vi "Close.vi"(8 "error in (no error)":errorcluster, 11 "Inst.FP in":refnum<class "Inst.FP.lvclass">) -> (0 "error out":errorcluster, 3 "Inst.FP out":refnum<class "Inst.FP.lvclass">)   [LabVIEW 2019, in "Inst.FP.lvclass"]
uses:
  Inst.FP.lvclass
  <userlib>/LevyLab/Instrument Framework/Instrument/Instrument.lvclass
  <userlib>/LevyLab/Instrument Framework/Instrument Types/Cryostat/Instrument.Cryostat.lvclass
  C:/Program Files (x86)/National Instruments/LabVIEW 2019/user.lib/LevyLab/Instrument Framework/Instrument Types/Cryostat/Instrument.Cryostat.lvclass
  C:/Program Files (x86)/National Instruments/LabVIEW 2019/user.lib/LevyLab/Instrument Framework/Instrument/Instrument.lvclass
  C:/Program Files (x86)/National Instruments/LabVIEW 2019/vi.lib/JKI/JKI SMO/SMO/SMO.lvclass
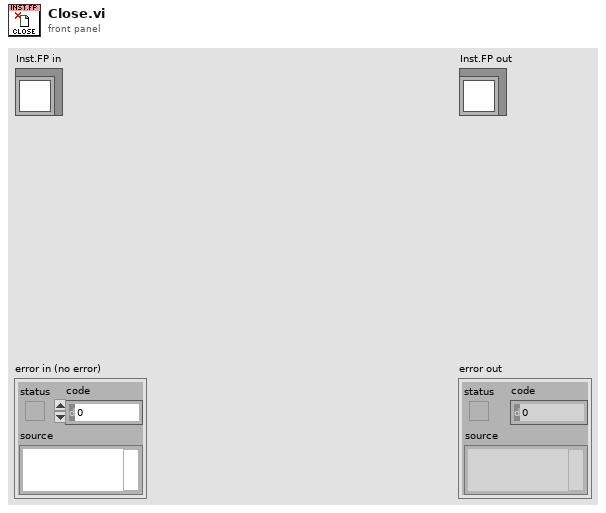
[diagram p1: front panel]
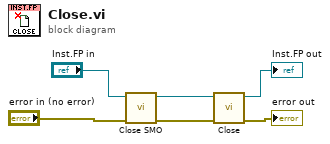
[diagram p0: block diagram]
diagram:
  n1 = call <userlib>:"Close SMO.vi"("error in (no error)"="error in (no error)", "Instrument in"="Inst.FP in") -> ("error out"=w2:errorcluster, "Instrument out"=w4:refnum<class "Inst.FP.lvclass">)  [unwired: 8 in]
  n2 = call-parent "Close.vi"("error in (no error)"=w2, "Instrument in"=w4) -> ("error out"=→"error out":errorcluster, "Instrument out"=→"Inst.FP out":refnum<class "Inst.FP.lvclass">)  [unwired: 8 in]
